vi "FTW-Reflection-Enum.vi"(7 "Enum":variant) -> (6 "Enum Items":string[](array[string]), 8 "Number of Items":i32, 10 "Selected Item":string)   [LabVIEW 2015]
panel:
  # "Inputs"
  # "Outputs"
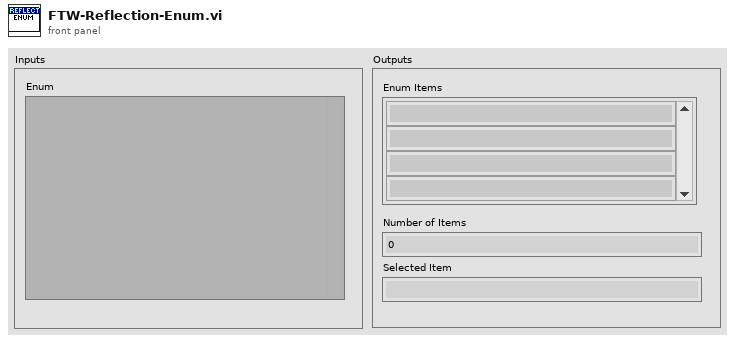
[diagram p1: front panel]
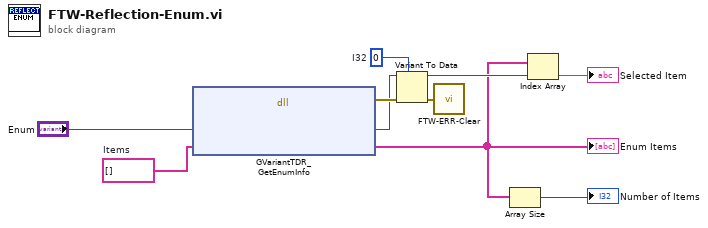
[diagram p0: block diagram]
diagram:
  w9 = 0  # I32
  w10 = string[] []  # Items
  n1 = dll-call lib="LabVIEW" fn="GVariantTDR_GetEnumInfo"("Input Enum Variant"="Enum", "Enum Items"=w10) -> (error out=w3:errorcluster, "Input Enum Variant"=w2:variant, "Enum Items"=w5:string[])  [unwired: 4 in, 1 out]
  "Enum Items" <- w5
  n2 = Variant To Data(error in=w3, type=w9, Variant=w2) -> (data=w7:i32, error out=w1:errorcluster)
  n3 = call "FTW-ERR-Clear.vi"("error to snuff"=w1) -> ()  [unwired: 1 out]
  n4 = Array Size(array=w5) -> (size(s)=→"Number of Items":i32)
  n5 = Index Array(array=w5, index=w7) -> (element=→"Selected Item":string)
